vi "CAN Frame to Table.vi"(7 "Hexadecimal?":bool, 8 "error in (no error)":errorcluster, 10 "CAN Frames (from XNET Read)":T1[](array[typedef]) {"payload" format="%x"; "timestamp" format="%<%.7X\n%x>T"; "type" items=["CAN Data"=0, "CAN Remote"=1, "CAN Bus Error"=2, "Delay"=224, "Log Trigger"=225, "Start Trigger"=226]; "identifier" format="%x"}, 11 "Input Array":string[][](array[string])) -> (0 "error out":errorcluster, 3 "Output Array":string[][](array[string]))   [LabVIEW 2013]
uses:
  <vilib>/xnet/xnet.llb/XNET Frame CAN.ctl
  <vilib>/xnet/xnet.llb/XNET Frame Type CAN.ctl
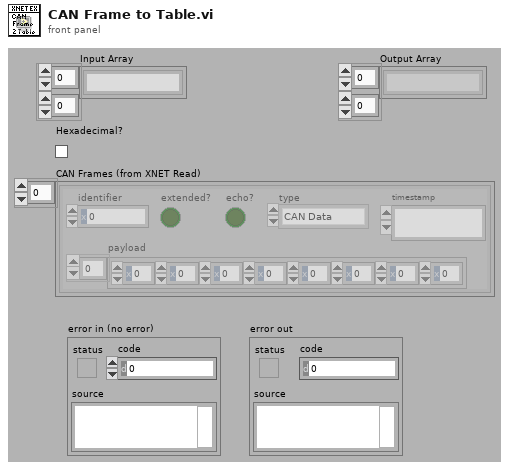
[diagram p1: front panel]
types:
  T1 = typedef "XNET Frame CAN.ctl" = cluster{"timestamp":timestamp, "payload":u8[], "identifier":u32, "type":T2, "extended?":bool, "echo?":bool}
  T2 = typedef "XNET Frame Type CAN.ctl" = u8
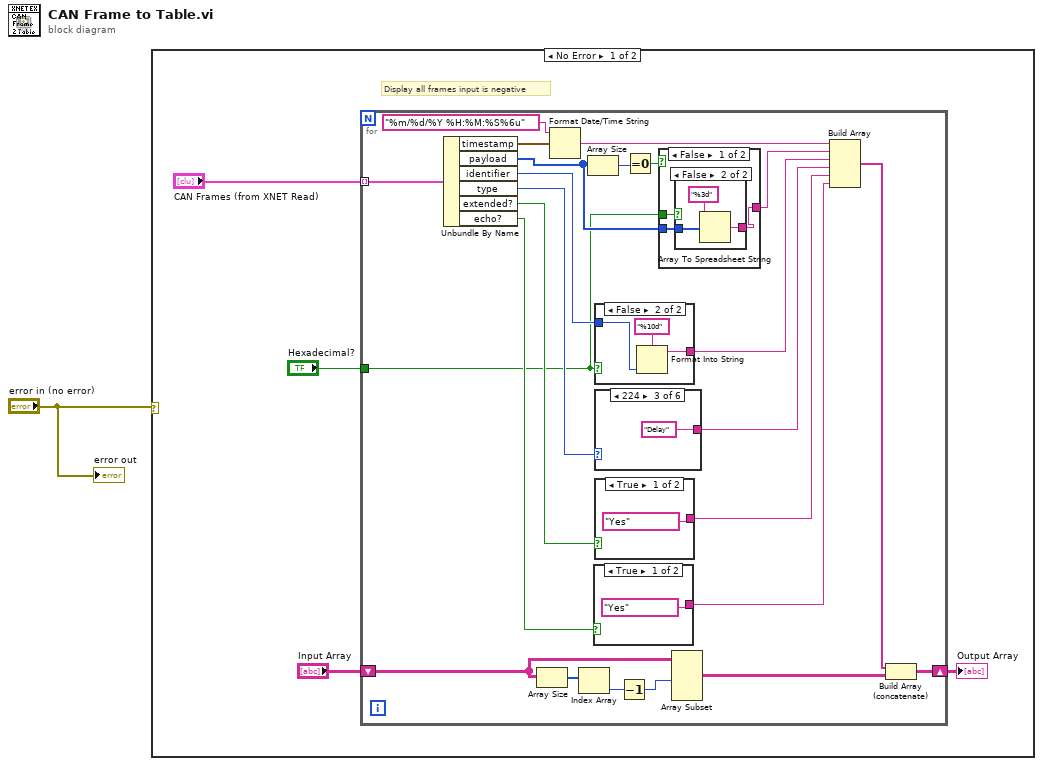
[diagram p0: block diagram]
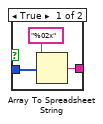
[diagram p2: hidden frame]
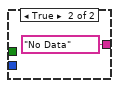
[diagram p3: hidden frame]
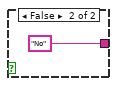
[diagram p4: hidden frame]
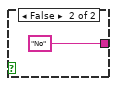
[diagram p5: hidden frame]
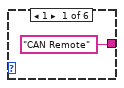
[diagram p6: hidden frame]
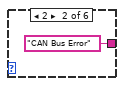
[diagram p7: hidden frame]
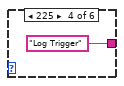
[diagram p8: hidden frame]
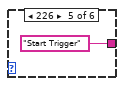
[diagram p9: hidden frame]
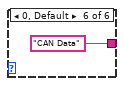
[diagram p10: hidden frame]
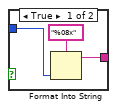
[diagram p11: hidden frame]
diagram:
  n1 = case shown="No Error" "error in (no error)" {
    frame No Error {
      # "Display all frames input is negative"
      n2 = for {
        tunnel: "CAN Frames (from XNET Read)" -> [w29] mode=indexing
        tunnel: "Hexadecimal?" -> [w13]
        shift-right: [w24] -> w3
        shift-left: "Input Array" -> [w7]
        n3 = Unbundle By Name(w29) -> ("timestamp"=w28:timestamp, "payload"=w14:u8[], "identifier"=w26:u32, "type"=w22:T2, "extended?"=w19:bool, "echo?"=w18:bool)
        n4 = Array Size(array=w7) -> (size(s)=w10:i32[])
        n5 = Format Date/Time String(time format string (%c)="%m/%d/%Y %H:%M:%S%6u", seconds (now)=w28) -> (date/time string=w27:string)  [unwired: 1 in]
        n6 = Index Array(array=w10) -> (element=w9:i32)  [unwired: 1 in]
        n7 = Array Size(array=w14) -> (size(s)=w17:i32)
        n8 = case shown="True" w18 {
          tunnel: ["Yes" "No"] -> w12
          frame True {
          }
          frame False {
          }
        }
        n9 = case shown="False" w13 {
          tunnel: w26 -> [w51 w54]
          tunnel: [w50 w53] -> w23
          frame True {
            n10 = Format Into String(format string="%08x", w51) -> (resulting string=w50:string)  [unwired: 2 in, 1 out]
          }
          frame False {
            n11 = Format Into String(format string="%10d", w54) -> (resulting string=w53:string)  [unwired: 2 in, 1 out]
          }
        }
        n12 = case shown="224" w22 {
          tunnel: ["CAN Remote" "CAN Bus Error" "Delay" "Log Trigger" "Start Trigger" "CAN Data"] -> w21
          frame 1 {
          }
          frame 2 {
          }
          frame 224 {
          }
          frame 225 {
          }
          frame 226 {
          }
          frame 0, Default {
          }
        }
        n13 = case shown="True" w19 {
          tunnel: ["Yes" "No"] -> w20
          frame True {
          }
          frame False {
          }
        }
        n14 = Decrement(x=w9) -> (x-1=w8:i32)
        n15 = Equal To 0?(x=w17) -> (x = 0?=w16:bool)
        n16 = case shown="False" w16 {
          tunnel: [w30 "No Data"] -> w15
          tunnel: w14 -> [w32 _]
          tunnel: w13 -> [w31 _]
          frame False {
            n17 = case shown="False" w31 {
              tunnel: w32 -> [w34 w37]
              tunnel: [w33 w36] -> w30
              frame True {
                n18 = Array To Spreadsheet String(array=w34, 3:"%02x" ("format string")) -> (spreadsheet string=w33:string)  [unwired: 1 in]
              }
              frame False {
                n19 = Array To Spreadsheet String(array=w37, 3:"%3d" ("format string")) -> (spreadsheet string=w36:string)  [unwired: 1 in]
              }
            }
          }
          frame True {
          }
        }
        n20 = Array Subset(array=w7, length (row)=w8) -> (w6:string[][])  [unwired: 3 in]
        n21 = Build Array(w27, w15, w23, w21, w20, w12) -> (w25:string[])
        n22 = Build Array (concatenate)(w25, w6) -> (w24:string[][])
      }
      "Output Array" <- w3
    }
    frame Error {
    }
  }
  "error out" <- "error in (no error)"
